vi "LoadModelList.vi"(7 "base path":path, 10 "Value":u16, 11 "Strings []":string[](array[string])) -> (2 "Model Strings":string[](array[string]))   [LabVIEW 2023, in "Configuration.lvlib" / "Configuration.lvclass"]
uses:
  Library/Configuration.lvclass
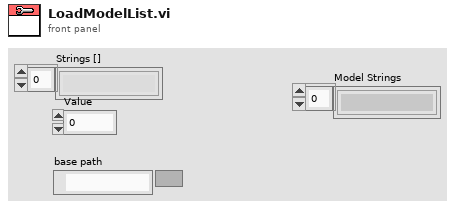
[diagram p1: front panel]
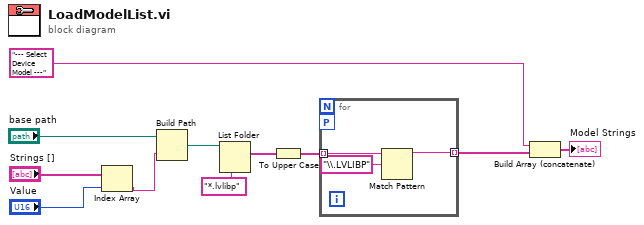
[diagram p0: block diagram]
diagram:
  n1 = Index Array(array="Strings []", index="Value") -> (element=w5:string)
  n2 = Build Path(base path="base path", name or relative path=w5) -> (appended path=w9:path)
  n3 = List Folder(path=w9, pattern="*.lvlibp") -> (filenames=w4:string[])  [unwired: 2 in, 3 out]
  n4 = To Upper Case(1:w4) -> (0:w3:string[])
  n5 = for {
    workers-P: _ -> [_]
    tunnel: w3 -> [w14] mode=indexing
    tunnel: [w12] -> w2 mode=indexing
    n6 = Match Pattern(string=w14, regular expression="\\.LVLIBP") -> (before substring=w12:string)  [unwired: 1 in, 3 out]
  }
  n7 = Build Array (concatenate)("--- Select Device Model ---", w2) -> (→"Model Strings":string[])
